vi "Find Event Frame.vi"(8 "error in":errorcluster, 9 "Broadcast?":bool, 10 "VI in":refnum<vi>, 11 "Application Instance":refnum<vi>) -> (0 "error out":errorcluster)   [LabVIEW 2019, in "Panther Dashboard.lvlib"]
uses:
  Panther Dashboard.lvlib
  <vilib>/Utility/traverseref.llb/TRef TravTarget.ctl
  <vilib>/Utility/traverseref.llb/VI Scripting - Traverse.lvlib
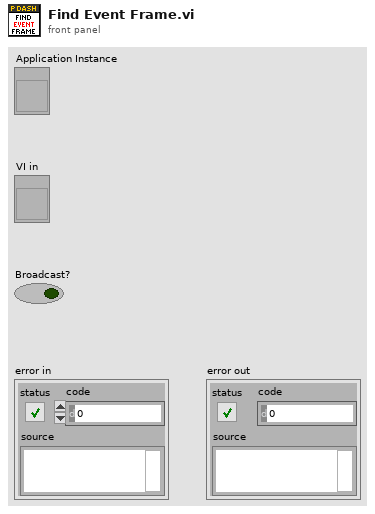
[diagram p1: front panel]
types:
  T1 = typedef "TRef TravTarget.ctl" = enum16{"FP", "BD", "Other"}
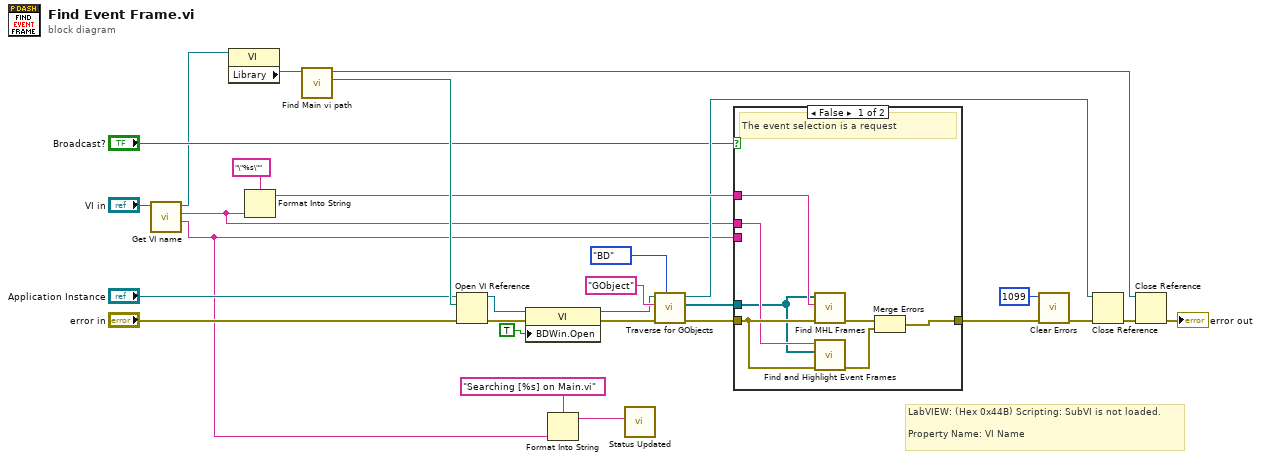
[diagram p0: block diagram]
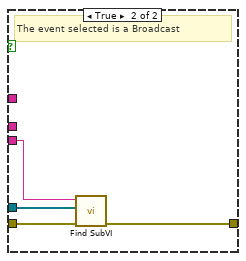
[diagram p2: hidden frame]
diagram:
  # "LabVIEW: (Hex 0x44B) Scripting: SubVI is not loaded.\n\nProperty Name: VI Name"
  n1 = call "Get VI name.vi"("VI in"="VI in") -> ("Full Vi Name"=w3:string, "Plain Name"=w7:string, "VI out"=w5:refnum<vi>)  [unwired: 8 in]
  n2 = property class="VI"(reference=w5) -> ("Library"=w6:refnum<vi>)  [unwired: 1 in, 2 out]
  n3 = Format Into String(format string="\"%s\"", w7) -> (resulting string=w16:string)  [unwired: 2 in, 1 out]
  n4 = call "Find Main vi path.vi"("Library in"=w6) -> ("Main vi Path"=w20:path, "Library out"=w18:refnum<vi>)  [unwired: 9 in]
  n5 = Open VI Reference(application reference (local)="Application Instance", vi path=w20, error in (no error)="error in") -> (vi reference=w19:refnum<vi>, error out=w29:errorcluster)  [unwired: 3 in]
  n6 = property class="VI"(reference=w19, error in=w29, "BDWin.Open"=TRUE ("Block Diagram Window:Open")) -> (reference out=w12:refnum<vi>, error out=w28:errorcluster)
  n7 = Format Into String(format string="Searching [%s] on Main.vi", w3) -> (resulting string=w4:string)  [unwired: 2 in, 1 out]
  n8 = call "Status Updated.vi"("Status"=w4) -> ()  [unwired: 10 in, 1 out]
  n9 = call <vilib>:"Traverse for GObjects.vi"("Traverse Target"=TRef_TravTarget."BD", "error in (no error)"=w28, "Class Name"="GObject", "VI Refnum"=w12) -> ("error out"=w27:errorcluster, "References"=w11:refnum<vi>[], "dup VI Refnum"=w10:refnum<vi>)  [unwired: 4 in, 1 out]
  n10 = case shown="False" "Broadcast?" {
    tunnel: w16 -> [w32 _]
    tunnel: w27 -> [w36 w40]
    tunnel: w11 -> [w30 w37]
    tunnel: w3 -> [_ w38]
    tunnel: w7 -> [w31 _]
    tunnel: [w34 w39] -> w23
    frame False {
      # "The event selection is a request"
      n11 = call "Find MHL Frames.vi"("error in"=w36, "Event Name"=w32, "References"=w30) -> ("error out"=w35:errorcluster)  [unwired: 8 in]
      n12 = call "Find and Highlight Event Frames.vi"("error in"=w36, "References"=w30, "Event Name"=w31) -> ("error out"=w33:errorcluster)  [unwired: 8 in]
      n13 = Merge Errors(w35, w33) -> (w34:errorcluster)
    }
    frame True {
      # "The event selected is a Broadcast"
      n14 = call "Find SubVI.vi"("error in"=w40, "References"=w37, "Full Vi Name"=w38) -> ("error out"=w39:errorcluster)  [unwired: 8 in]
    }
  }
  n15 = call <vilib>:"Clear Errors.vi"("error in (no error)"=w23, "specific error code to clear (0: all)"=1099) -> ("error out"=w22:errorcluster)  [unwired: 4 in, 1 out]
  n16 = Close Reference(reference=w10, error in (no error)=w22) -> (error out=w25:errorcluster)
  n17 = Close Reference(reference=w18, error in (no error)=w25) -> (error out=→"error out":errorcluster)
